vi "S2C_ResetPanel.vi"(8 "Error In":errorcluster) -> (0 "Error Out":errorcluster)   [LabVIEW 2015]
doc: "Initializes all front panel controls to their default states."
uses:
  Globals/S2C_Globals.vi
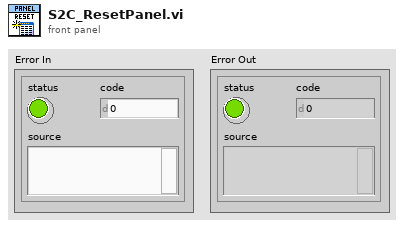
[diagram p1: front panel]
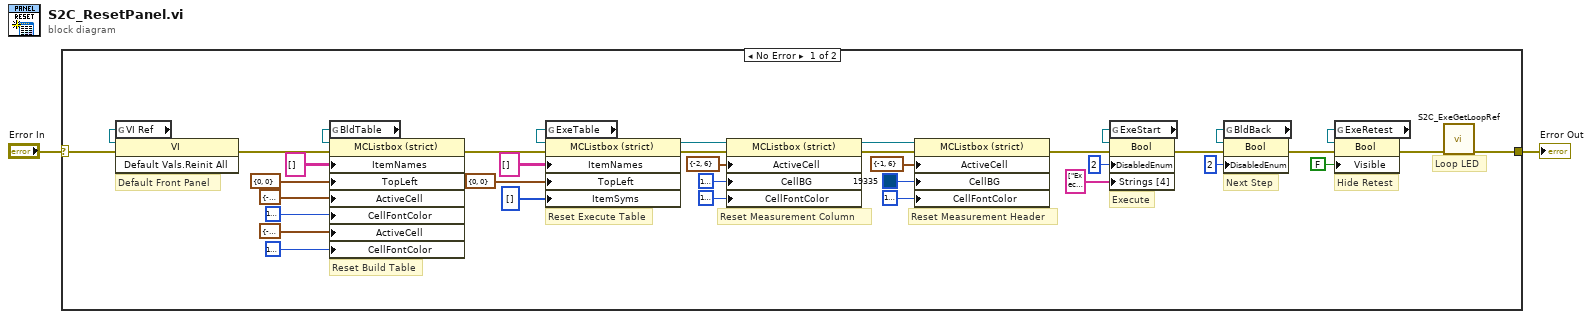
[diagram p0: block diagram]
diagram:
  n1 = case shown="No Error" "Error In" {
    selector: "Error In" -> [w39 w40]
    tunnel: [w9 w40] -> w1
    frame No Error {
      # "Hide Retest"
      # "Loop LED"
      # "Next Step"
      # "Reset Execute Table"
      # "Execute"
      # "Reset Measurement Header"
      # "Reset Measurement Column"
      # "Reset Build Table"
      # "Default Front Panel"
      n2 = global read "S2C_Globals.vi" "VI Ref"() -> (w16:refnum<vi>)
      n3 = invoke class="VI" method="Default Vals.Reinit All"(reference=w16, error in=w39) -> (error out=w36:errorcluster)  [unwired: 1 in, 2 out]
      n4 = global read "S2C_Globals.vi" "BldTable"() -> (w35:refnum<vi>)
      n5 = property class="MCListbox (strict)"(reference=w35, error in=w36, "ItemNames"=string[][] [] ("Item Names"), "TopLeft"=cluster{"Row":u32, "Column":u32} {"Row"=0, "Column"=0} ("Top Left Visible Cell"), "ActiveCell"=cluster{"Row":i32, "Column":i32} {"Row"=-2, "Column"=-2} ("Active Cell:Active Cell"), "CellFontColor"=u32 16777222, "ActiveCell"=cluster{"Row":i32, "Column":i32} {"Row"=-1, "Column"=-2} ("Active Cell:Active Cell"), "CellFontColor"=u32 16777226) -> (error out=w23:errorcluster)  [unwired: 1 out]
      n6 = global read "S2C_Globals.vi" "ExeTable"() -> (w21:refnum<vi>)
      n7 = property on="Property Node" class="MCListbox (strict)"(reference=w21, error in=w23, "ItemNames"=string[][] [] ("Item Names"), "TopLeft"=cluster{"Row":u32, "Column":u32} {"Row"=0, "Column"=0} ("Top Left Visible Cell"), "ItemSyms"=i32[] [] ("Item Symbols")) -> (reference out=w33:refnum<vi>, error out=w30:errorcluster)
      n8 = property on="Property Node" class="MCListbox (strict)"(reference=w33, error in=w30, "ActiveCell"=cluster{"Row":i32, "Column":i32} {"Row"=-2, "Column"=6} ("Active Cell:Active Cell"), "CellBG"=u32 16777226, "CellFontColor"=u32 16777222) -> (reference out=w34:refnum<vi>, error out=w24:errorcluster)
      n9 = property on="Property Node" class="MCListbox (strict)"(reference=w34, error in=w24, "ActiveCell"=cluster{"Row":i32, "Column":i32} {"Row"=-1, "Column"=6} ("Active Cell:Active Cell"), "CellBG"=u32 19335, "CellFontColor"=u32 16777226) -> (error out=w19:errorcluster)  [unwired: 1 out]
      n10 = global read "S2C_Globals.vi" "ExeStart"() -> (w18:refnum<vi>)
      n11 = property class="Bool"(reference=w18, error in=w19, "DisabledEnum"=u8 2, "Strings [4]"=string[] ["Execute Script", "Abort Testing"] ("Array - String")) -> (error out=w7:errorcluster)  [unwired: 1 out]
      n12 = global read "S2C_Globals.vi" "BldBack"() -> (w11:refnum<vi>)
      n13 = property class="Bool"(reference=w11, error in=w7, "DisabledEnum"=u8 2) -> (error out=w4:errorcluster)  [unwired: 1 out]
      n14 = global read "S2C_Globals.vi" "ExeRetest"() -> (w6:refnum<vi>)
      n15 = property class="Bool"(reference=w6, error in=w4, "Visible"=FALSE) -> (error out=w3:errorcluster)  [unwired: 1 out]
      n16 = call "S2C_ExeGetLoopRef.vi"("Error In"=w3) -> ("Error Out"=w9:errorcluster)  [unwired: 10 in]
    }
    frame Error {
    }
  }
  "Error Out" <- w1
